vi "AppInit.vi"(10 "path":path, 11 "Changelog":string caption="App Ver") -> (0 "error out":errorcluster)   [LabVIEW 2016]
doc: "Init Host application"
uses:
  tools/Windows/Windows.ExitAction.ctl
  tools/EventLog/EventLog.Buffer.Action.ctl
  tools/Translator/Translator.Message.ctl
  Global/ApplicationGlobal.vi
  tools/EventLog/EventLog.New(single).vi
panel:
  out "idx":i32
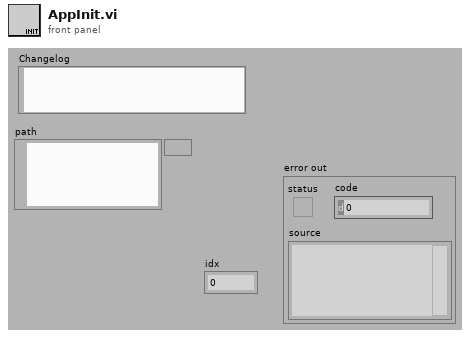
[diagram p1: front panel]
types:
  T1 = typedef "Windows.ExitAction.ctl" = enum16{"Log off from PC", "Shut Down PC", "Reboot PC", "Close Program"}
  T2 = typedef "EventLog.Buffer.Action.ctl" = enum16{"init", "re-init", "clear", "set translator", "add", "get", "get unsaved"}
  T3 = typedef "Translator.Message.ctl" = enum16{"-", "Event confirmed", "Log out", "Log in", "Shutdown", "Cancel", "Start", "Begin time", "End time", "Duration", "Service Mode", "Ignore Results", "Serial Format", "On", "Off", "OK", "NOK", "NOK %s", "Home", "Work", "Close", "Open", "In progress...", "Missing", "Empty", "Hardware failure", "Initial", "Default", "Total", "Out of range", "Free disk space is below 1GB - contact technician", "Error %d >> %s", "Error %d >> %s >> %s", "Msg %d >> %s", "Laser msg %d %s", "Laser cmd error %s %d", "Laser cmd failed %s", "Laser cmd warning %s", "Laser disconnected", "Laser status %s", "Laser already started", "Laser job unkonwn %s", "Laser job missing %s", "Laser job select failure %s", "Unable to start laser printing (%s)", "Unable to stop laser printing (%s)", "Laser marking aborted", "Laser marking timeout", "Unable to reset Laser Interlock (%s)", "Unable to trigger Laser. Laser not ready (%s)", "Laser job '%s' coordinates not configured", "Starting %s", "Quitting %s", "Configured", "Initializing", "Quitting", "Loading", "Loaded %d results", "Loaded %d events", "Running", "Stopped", "Summary", "Laser", "Do you want to continue?", "Do you want to delete the configuration?", "The configuration is being used by an order. Unable to delete!", "Press confirm button", "Station is not based. Do you want to exit?", "Station requires changeover. Do you want to run the test?", "Test options are not set as default. Do you want to continue?", "Formatting of WabcoNo is disabled. Do you want to continue?", "Product not detected. Do you want to continue?", "Product scan failed. Do you want to continue?", "Calibration", "Log out?", "System", "All", "IDLE", "Translating...%s", "Not found", "Alarm %s", "Run", "Skip", "Abort", "Repeat", "Please wait...", "Database disconnected", "Database disconnected - changeover disabled!", "Login to database successful", "Login to database failed: %d; %s", "Unable to check the product status of reference %d - database disconnected", "Unable to set the product status of reference %d - database disconnected", "Variant file backup %s", "Read variant (%s)", "Result", "Station armed!", "Station requires changeover!", "Select reference number...", "EMERGENCY BUTTON - press Control button", "EMERGENCY DOOR - press Control button", "Resetting Emergency...", "Unable to reset safety circuit - Emergency Button pressed", "Unable to reset safety circuit - Emergency Side Door open", "Station not based", "Station based", "Station not empty", "Station basing...", "No order", "Press Start to begin new order", "Scanning new order", "Order NOK. Correct or scan again", "Order OK. Press Accept", "Order ready", "Revolver incorrect", "Fork incorrect", "Revolver missing", "Revolver empty", "Container missing", "Offline results", "Offline statistics", "Updating statistics %.1f %%", "DMC Configurator", "Door open", "Close the front door", "Press start button", "Done. Open the front door", "Running...", "Running...%.1f %%", "Pause %s", "Pause %s. NOK container missing", "Pause %s. OK container missing", "Pause %s. Revolver empty", "Pause %s. Revolver missing", "Pause %s. Revolver incorrect", "Pause %s. Fork missing", "Pause %s. Fork incorrect", "Pause %s. Too many failures", "Pause %s. Unloading failure", "Pause %s. One slot is not working", "Pause %s. Part order is done. Empty OK container", "Pause %s. Unable to move product to slot", "Pause %s. Unable to move back product pusher", "Pause %s. Unable to lift product", "Pause %s. Unable to move back product lifter", "Pause %s. Unable to move product arm to Work", "Pause %s. Unable to move product arm to NOK", "Pause %s. Unable to move product arm to OK", "Pause %s. Unable to unsuck the NOK product", "Pause %s. Unable to drop the NOK product", "Pause %s. Product OK missing", "Pause %s. Unable to unsuck the OK product", "Pause %s. Unable to drop the OK product", "Stopping...", "File '%s' is missing", "File '%s' is broken", "File '%s' is running", "Log file started (%s)", "Log file ended (%s)", "Log file stopped (%s)", "Log file ignored (%s)", "Log file exported (%s)", "Log file export failed (%s)", "Wrong serial number in log file", "Wrong reference number in log file", "Test steps are missing", "%s = %.3f", "Process param '%s' not found in DB", "Process param '%s' wrong order", "Process param '%s' value %.3f out of limits (%.3f; %.3f)", "Step%d param '%s' not found in DB", "Step%d param '%s' wrong order", "Step%d param '%s' value %.3f out of limits (%.3f; %.3f)", "Step%d EV '%s' not found in DB", "Step%d EV '%s' wrong order", "\"%s\" not found in DB", "\"%s\" wrong order", "\"%s\" value %.3f out of limits (%.3f; %.3f)", "\"%s\" not found in software", "Process init (%s)", "Process started", "Process restarted", "Process run", "Process done", "Process done - remove OK container", "Process aborted", "Process aborted at work", "Process aborted at home", "Process error", "Process error at home", "Process error at work", "Process close", "Process pause", "Process continue", "Process door open", "Process door close", "Process pause at slot %s due to %s", "Select plate from the order to process", "Do you want to start the process?", "Do you want to continue the process?", "There is unfinished order. Do you want to put the new order?", "Product %s %d OK", "Product %s %d NOK", "Unable to unload the slot %s. Product missing in the slot", "Unable to unload the slot %s. Product already in the arm", "Unable to accept the product as OK. Product missing in slot %s", "Unable to accept the product as OK. Product could not drop into the container at slot %s", "Unable to accept the product as NOK. Product could not drop into the container at slot %s", "Scan failed. Error %s", "Scan failed. Scanner disconnected", "Scan failed. Wrong Wabco number %d, limit (%d,%d)", "Scan failed. Wrong serial number %d, limit (%d,%d)", "Scan failed. Wrong date %d, limit (%d,%d)", "Scan failed. Wrong product wabco number %d (expected %d)", "Scan failed. Wrong product serial number %d (expected > 0)", "Scan OK %s", "Scan failed. Unable to determine table position (%s)", "Scan failed. Timeout", "Tune failed. Scanner disconnected", "Tune failed. Timeout", "%s = %d", "%s = %d->%d", "Unable to set %s = %.2f - Air Pressure Inside off", "Unable to set digital output '%s' = %d", "Unable to activate air pressure inside - timeout", "Unable to activate air pressure inside - aborted", "Unable to switch on Air Main Valve - Air Pressure Inlet off", "Unable to switch on Air Main Valve - Door open", "Unable to switch off Air Main Valve - timeout", "Unable to switch off Air Main Valve - aborted", "Unable to rotate Table - timeout", "Unable to rotate Table - aborted", "Unable to rotate Table - Product Move not in Home position", "Unable to rotate Table - Air Pressure Inside off", "Unable to rotate Table - Product Lift A not in Home position", "Unable to rotate Table - Product Lift B not in Home position", "Unable to rotate Table - unlock before movement timeout", "Unable to rotate Table - lock after movement timeout", "Unable to move Table Lock to %s position - timeout", "Unable to move Table Lock to %s position - aborted", "Unable to move Table Lock to %s position - Air Pressure Inside off", "Unable to move Table Lock to %s position - Table not in position", "Unable to move Product Lift A to %s position - timeout", "Unable to move Product Lift B to %s position - timeout", "Unable to move Product Lift A to %s position - aborted", "Unable to move Product Lift B to %s position - aborted", "Unable to move Product Lift A to %s position - Air Pressure Inside off", "Unable to move Product Lift B to %s position - Air Pressure Inside off", "Unable to move Product Lift A to %s position - Table not locked", "Unable to move Product Lift B to %s position - Table not locked", "Unable to move Product Lift A to %s position - Product Arm not in Work position", "Unable to move Product Lift B to %s position - Product Arm not in Work position", "Unable to set Product Suction Gripper %s to %s - timeout", "Unable to set Product Suction Gripper %s to %s - aborted", "Unable to set Product Suction Gripper %s to %s - Air Pressure Inside off", "Unable to set Product Suction Gripper %s to %s - Table slot unkown", "Unable to move Product Arm to %s position - timeout", "Unable to move Product Arm to %s position - aborted", "Unable to move Product Arm to %s position - Air Pressure Inside off", "Unable to move Product Arm to %s position - Product Lift A not in Home position", "Unable to move Product Arm to %s position - Product Lift B not in Home position", "Unable to move Product to %s position - timeout", "Unable to move Product to %s position - aborted", "Unable to move Product to %s position - Air Pressure Inside off", "Unable to move Product to %s position - Table not in position"}
  T4 = enum32{"invalid app kind", "Development System", "Run Time System", "Student Edition", "Embedded LabVIEW", "Evaluation", "Custom"}
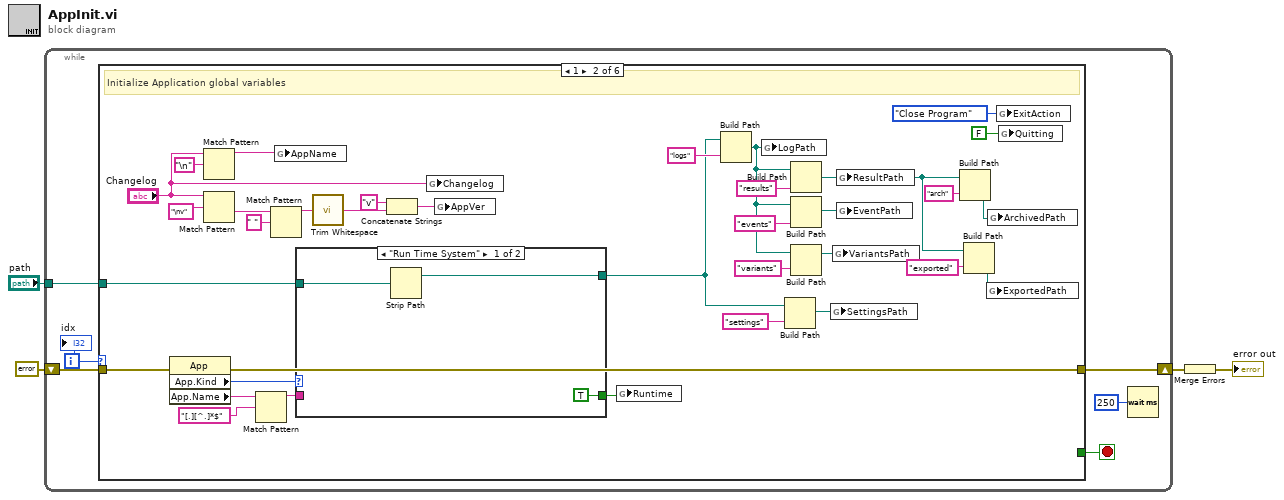
[diagram p0: block diagram]
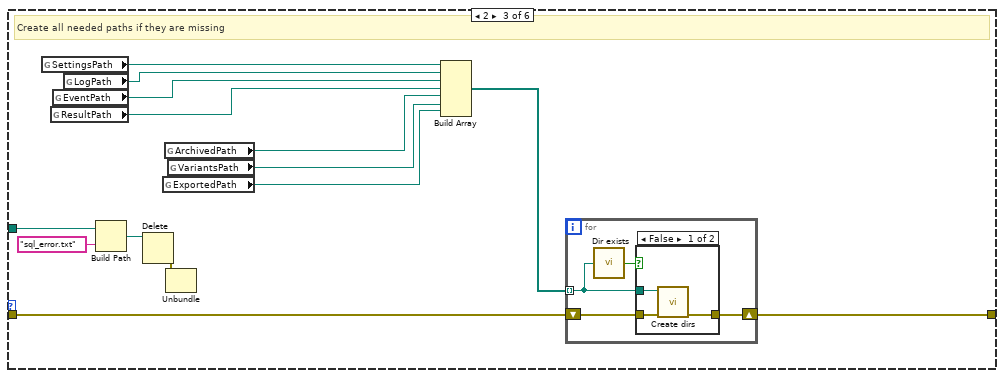
[diagram p4: hidden frame]
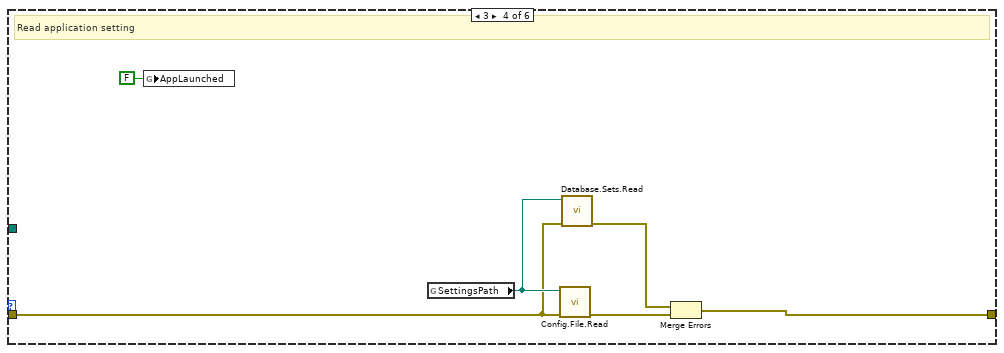
[diagram p6: hidden frame]
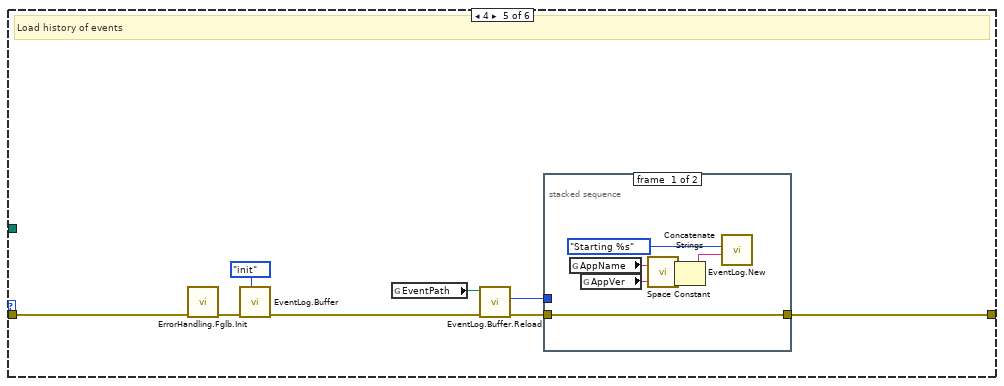
[diagram p7: hidden frame]
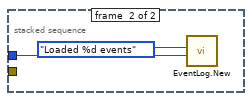
[diagram p8: hidden frame]
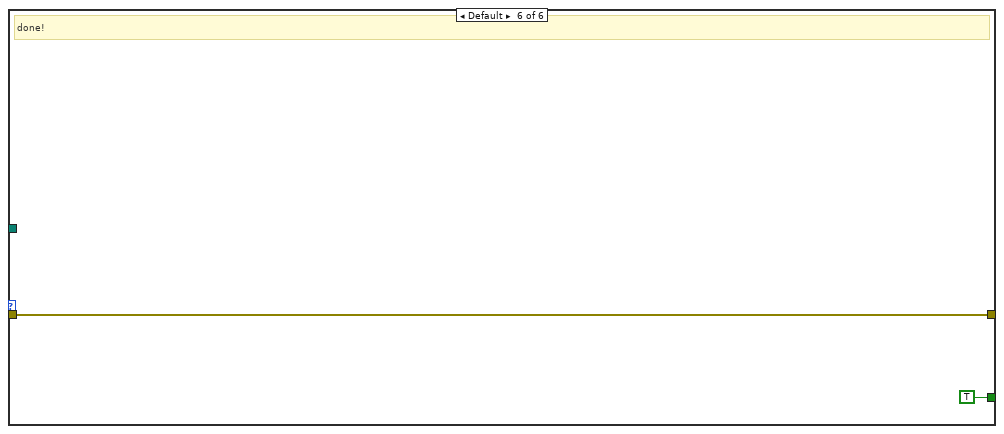
[diagram p9: hidden frame]
diagram:
  n1 = while {
    shift-right: [w8] -> w3
    shift-left: errorcluster {"status"=FALSE, "code"=0, "source"=""} ("error out") -> [w10]
    tunnel: "path" -> [w7]
    i -> [w6]
    stop <- w9 stop-if-true
    n2 = case shown="1" w6 {
      tunnel: w10 -> [w11 w12 w51 w73 w79 w95]
      tunnel: [_ _ _ _ _ TRUE] -> w9
      tunnel: [w11 w13 w62 w74 w84 w95] -> w8
      tunnel: w7 -> [_ w28 w58 _ _ _]
      frame 0 {
        # "Hide top level VI (Main.vi) panel"
      }
      frame 1 {
        # "Initialize Application global variables"
        n3 = property class="App"(error in=w12) -> (error out=w13:errorcluster, "App.Kind"=w38:T4, "App.Name"=w32:string)  [unwired: 1 in, 1 out]
        n4 = Match Pattern(string="Changelog", regular expression="\n") -> (before substring=w27:string)  [unwired: 1 in, 3 out]
        n5 = Match Pattern(string="Changelog", regular expression="\nv") -> (after substring=w44:string)  [unwired: 1 in, 3 out]
        n6 = Match Pattern(string=w32, regular expression="[.][^.]*$") -> (before substring=w31:string)  [unwired: 4 out]
        n7 = Match Pattern(string=w44, regular expression=" ") -> (before substring=w41:string)  [unwired: 1 in, 3 out]
        n8 = global write "ApplicationGlobal.vi" "AppName"(w27) -> ()
        n9 = case shown="\"Run Time System\"" w38 {
          tunnel: [w49 w50] -> w25
          tunnel: w31 -> [_ _]
          tunnel: w28 -> [w48 w50]
          tunnel: [TRUE ("Quitting") _] -> w22
          frame "Run Time System" {
            n10 = Strip Path(path=w48) -> (stripped path=w49:path)  [unwired: 1 out]
          }
          frame Default {
          }
        }
        n11 = call <vilib>:"Trim Whitespace.vi"("string"=w41) -> ("trimmed string"=w39:string)  [unwired: 1 in]
        n12 = Concatenate Strings("v" ("string"), w39) -> (w26:string)
        n13 = global write "ApplicationGlobal.vi" "Changelog"("Changelog") -> ()
        n14 = global write "ApplicationGlobal.vi" "AppVer"(w26) -> ()
        n15 = global write "ApplicationGlobal.vi" "Runtime"(w22) -> ()
        n16 = Build Path(base path=w25, name or relative path="logs") -> (appended path=w16:path)
        n17 = global write "ApplicationGlobal.vi" "LogPath"(w16) -> ()
        n18 = Build Path(base path=w25, name or relative path="settings") -> (appended path=w24:path)
        n19 = Build Path(base path=w16, name or relative path="results") -> (appended path=w19:path)
        n20 = Build Path(base path=w16, name or relative path="events") -> (appended path=w35:path)
        n21 = Build Path(base path=w16, name or relative path="variants") -> (appended path=w14:path)
        n22 = global write "ApplicationGlobal.vi" "SettingsPath"(w24) -> ()
        n23 = global write "ApplicationGlobal.vi" "VariantsPath"(w14) -> ()
        n24 = global write "ApplicationGlobal.vi" "ResultPath"(w19) -> ()
        n25 = global write "ApplicationGlobal.vi" "EventPath"(w35) -> ()
        n26 = Build Path(base path=w19, name or relative path="arch") -> (appended path=w20:path)
        n27 = Build Path(base path=w19, name or relative path="exported") -> (appended path=w17:path)
        n28 = global write "ApplicationGlobal.vi" "ExportedPath"(w17) -> ()
        n29 = global write "ApplicationGlobal.vi" "ArchivedPath"(w20) -> ()
        n30 = global write "ApplicationGlobal.vi" "ExitAction"(Windows.ExitAction."Close Program" ("ExitAction")) -> ()
        n31 = global write "ApplicationGlobal.vi" "Quitting"(FALSE ("Quitting")) -> ()
      }
      frame 2 {
        # "Create all needed paths if they are missing"
        n32 = global read "ApplicationGlobal.vi" "SettingsPath"() -> (w56:path)
        n33 = global read "ApplicationGlobal.vi" "ResultPath"() -> (w55:path)
        n34 = global read "ApplicationGlobal.vi" "EventPath"() -> (w63:path)
        n35 = global read "ApplicationGlobal.vi" "LogPath"() -> (w64:path)
        n36 = Build Path(base path=w58, name or relative path="sql_error.txt") -> (appended path=w59:path)
        n37 = Delete(path (use dialog)=w59) -> (error out=w57:errorcluster)  [unwired: 4 in, 2 out]
        n38 = global read "ApplicationGlobal.vi" "ExportedPath"() -> (w52:path)
        n39 = global read "ApplicationGlobal.vi" "ArchivedPath"() -> (w54:path)
        n40 = Unbundle(w57) -> ()  [unwired: 3 out]
        n41 = global read "ApplicationGlobal.vi" "VariantsPath"() -> (w53:path)
        n42 = Build Array(w56, w64, w63, w55, w54, w53, w52) -> (w61:path[])
        n43 = for {
          tunnel: w61 -> [w66] mode=indexing
          shift-right: [w67] -> w62
          shift-left: w51 -> [w68]
          n44 = call "Dir exists.vi"("dir path"=w66) -> ("exists?"=w65:bool)  [unwired: 4 in]
          n45 = case shown="False" w65 {
            tunnel: w66 -> [w71 _]
            tunnel: w68 -> [w70 w72]
            tunnel: [w69 w72] -> w67
            frame False {
              n46 = call "Create dirs.vi"("error in (no error)"=w70, "deepest dir"=w71) -> ("error"=w69:errorcluster)  [unwired: 9 in]
            }
            frame True {
            }
          }
        }
      }
      frame 3 {
        # "Read application setting"
        n47 = global write "ApplicationGlobal.vi" "AppLaunched"(FALSE ("AppLaunched")) -> ()
        n48 = global read "ApplicationGlobal.vi" "SettingsPath"() -> (w76:path)
        n49 = call "Config.File.Read.vi"("error in"=w73, "path"=w76) -> ("error out"=w77:errorcluster)  [unwired: 9 in]
        n50 = call "Database.Sets.Read.vi"("error in"=w73, "SettingsPath"=w76) -> ("error out"=w75:errorcluster)  [unwired: 9 in]
        n51 = Merge Errors(w75, w77) -> (w74:errorcluster)
      }
      frame 4 {
        # "Load history of events"
        n52 = call "ErrorHandling.Fglb.Init.vi"("error in (no error)"=w79) -> ("error out"=w81:errorcluster)  [unwired: 10 in]
        n53 = call "EventLog.Buffer.vi"("action (get)"=EventLog.Buffer.Action."init" ("action (read)"), "error in"=w81) -> ("error out"=w82:errorcluster)  [unwired: 6 in, 3 out]
        n54 = global read "ApplicationGlobal.vi" "EventPath"() -> (w86:path)
        n55 = call "EventLog.Buffer.Reload.vi"("error in"=w82, "Path"=w86) -> ("error out"=w85:errorcluster, "#loaded entries"=w80:i32)  [unwired: 8 in]
        n56 = stacked-sequence {
          tunnel: [w91 _] -> w84
          tunnel: w85 -> [w91 _]
          tunnel: w80 -> [_ w93]
          frame #0 {
            n57 = global read "ApplicationGlobal.vi" "AppName"() -> (w90:string)
            n58 = global read "ApplicationGlobal.vi" "AppVer"() -> (w89:string)
            n59 = call <vilib>:"Space Constant.vi"() -> ("String"=w88:string)
            n60 = Concatenate Strings(w90, w88, w89) -> (w87:string)
            n61 = call-poly "EventLog.New.vi"("Arg"=w87, "Message (-)"=Translator.Message."Starting %s") -> ()  [unwired: 8 in, 2 out]
          }
          frame #1 {
            n62 = call-poly "EventLog.New.vi"("Arg"=w93, "Message (-)"=Translator.Message."Loaded %d events") -> ()  [unwired: 8 in, 2 out]
          }
        }
      }
      frame Default {
        # "done!"
      }
    }
    n63 = Wait (ms)(milliseconds to wait=u32 250) -> ()  [unwired: 1 out]
    "idx" <- w6
  }
  n64 = Merge Errors(w3) -> (→"error out":errorcluster)
